vi "getINI.vi"(7 "LVWSR":refnum<class "Web Request.lvclass">) -> ()   [LabVIEW 2014]
uses:
  <vilib>/wsapi/Web Request.lvclass
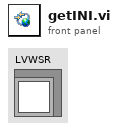
[diagram p1: front panel]
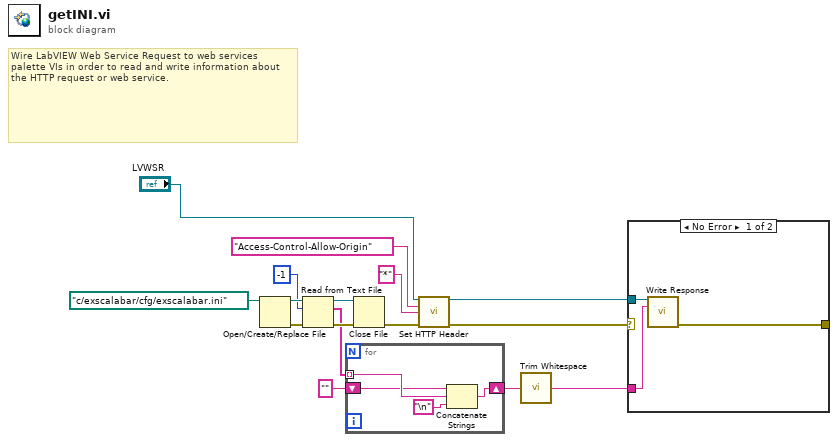
[diagram p0: block diagram]
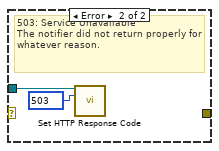
[diagram p2: hidden frame]
diagram:
  # "Wire LabVIEW Web Service Request to web services palette VIs in order to read and write information about the HTTP request or web service."
  n1 = Open/Create/Replace File(file path (use dialog)=path "c:/exscalabar/cfg/exscalabar.ini" ("Folder Path")) -> (refnum out=w11:refnum<file>, error out=w7:errorcluster)  [unwired: 5 in, 1 out]
  n2 = Read from Text File(file (use dialog)=w11, count=-1, error in=w7) -> (refnum out=w9:refnum<file>, text=w5:string[], error out=w10:errorcluster)  [unwired: 1 in, 1 out]
  n3 = for {
    tunnel: w5 -> [w20] mode=indexing
    shift-right: [w18] -> w3
    shift-left: "" -> [w19]
    n4 = Concatenate Strings(w19, w20, "\n") -> (w18:string)
  }
  n5 = Close File(refnum=w9, error in=w10) -> (error out=w8:errorcluster)  [unwired: 1 out]
  n6 = call <vilib>:"Set HTTP Header.vi"("LabVIEW Web Service Request"="LVWSR", "header"="Access-Control-Allow-Origin", "header value"="*", "error in (no error)"=w8) -> ("LabVIEW Web Service Request out"=w14:refnum<class "Web Request.lvclass">, "error out"=w13:errorcluster)  [unwired: 10 in]
  n7 = call <vilib>:"Trim Whitespace.vi"("string"=w3) -> ("trimmed string"=w2:string)  [unwired: 1 in]
  n8 = case shown="No Error" w13 {
    tunnel: w14 -> [w23 w25]
    tunnel: w2 -> [w22 _]
    tunnel: [w21 _] -> _
    frame No Error {
      n9 = call <vilib>:"Write Response.vi"("LabVIEW Web Service Request"=w23, "response string"=w22) -> ("error out"=w21:errorcluster)  [unwired: 12 in, 1 out]
    }
    frame Error {
      w24 = 503 items=["100"=100, "101"=101, "200"=200, "201"=201, "202"=202, "203"=203, "204"=204, "205"=205, "206"=206, "300"=300, "301"=301, "302"=302, "303"=303, "304"=304, "305"=305, "306"=306, "307"=307, "400"=400, "401"=401, "402"=402, "403"=403, "404"=404, "405"=405, "406"=406, "407"=407, "408"=408, "409"=409, "410"=410, "411"=411, "412"=412, "413"=413, "414"=414, "415"=415, "416"=416, "417"=417, "500"=500, "501"=501, "502"=502, "503"=503, "504"=504, "505"=505] ("response code (200)")
      # "503: Service Unavailable\nThe notifier did not return properly for whatever reason."
      n10 = call <vilib>:"Set HTTP Response Code.vi"("LabVIEW Web Service Request"=w25, "response code (200)"=w24) -> ()  [unwired: 12 in, 2 out]
    }
  }
